vi "Write Input Data.vi"(10 "Input Data":T1={"Limit Switches"={"1"=FALSE, "2"=FALSE}, "SSI Encoder"=0, "Force Measured"=0.0, "Distance Data"={"Distance Measured 1"=1.0, "Distance Measured 2"=1.0}, "Thermocouple Data"={"Motor Temperature"=274.15}} {"Thermocouple Data"."Motor Temperature" min=274.15 max=573.15 format="%.1f"; "Distance Data"."Distance Measured 2" min=1.0 max=300.0 format="%.1f"; "Distance Data"."Distance Measured 1" min=1.0 max=300.0 format="%.1f"; "Force Measured" min=-888.0 max=888.0 format="%.2f"}, 11 "Logger in":refnum<class "TestDataLog.lvclass">) -> (3 "Logger out":refnum<class "TestDataLog.lvclass">)   [LabVIEW 2013, in "TestDataLog.lvclass"]
uses:
  TestDataLog.lvclass
  Typedefs/InputData.ctl
  <userlib>/Common/ILC/Typedefs/LimitSwitches.ctl
  Typedefs/ForceDemand.ctl
  <userlib>/Common/Devices/DistanceGauge/Typedefs/Distance Data.ctl
  Typedefs/ThermocoupleData.ctl
  TestDataLog.lvclass/TestDataLog.ctl
  <userlib>/Common/ILC/Typedefs/ILCTypedefs.lvlib
  Typedefs/FAMTTypedefs.lvlib
  <userlib>/Common/Devices/DistanceGauge/DistanceGauge.lvlib
panel:
  # "Limit Switches"
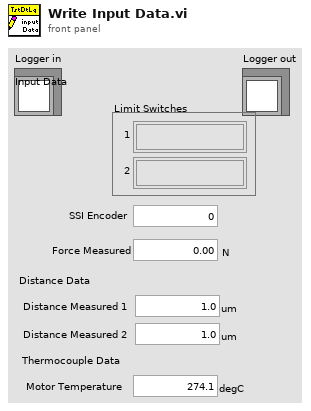
[diagram p1: front panel]
types:
  T1 = typedef "FAMTTypedefs.lvlib/InputData.ctl" = cluster{"Limit Switches":T2, "SSI Encoder":i32, "Force Measured":T3, "Distance Data":T4, "Thermocouple Data":T5}
  T2 = typedef "ILCCommon.lvlib/ILCTypedefs.lvlib/LimitSwitches.ctl" = cluster{"1":bool, "2":bool}
  T3 = typedef "FAMTTypedefs.lvlib/ForceDemand.ctl" = dbl[unit]
  T4 = typedef "DistanceGauge.lvlib/Distance Data.ctl" = cluster{"Distance Measured 1":dbl[unit], "Distance Measured 2":dbl[unit]}
  T5 = typedef "FAMTTypedefs.lvlib/ThermocoupleData.ctl" = cluster{"Motor Temperature":dbl[unit]}
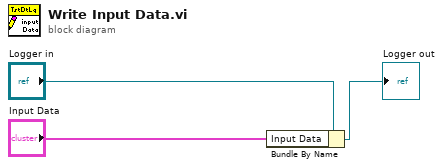
[diagram p0: block diagram]
diagram:
  n1 = Bundle By Name(cluster="Logger in", "Input Data"="Input Data") -> (→"Logger out":refnum<class "TestDataLog.lvclass">)
